vi "tpg361_visa_close.vi"(8 "error in (no error)":errorcluster, 11 "VISA session":refnum<visa-resource-name>) -> (0 "error out":errorcluster)   [LabVIEW 2019]
doc: "This VI closes the instrument.\n\nWARNINGS: \nYou MUSThave VISA Version 2.0 or higher installed to use this Instrument driver."
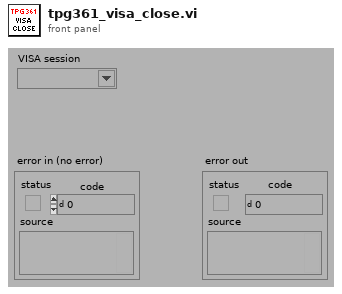
[diagram p1: front panel]
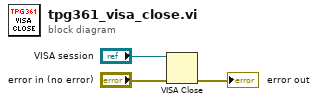
[diagram p0: block diagram]
diagram:
  n1 = VISA Close(VISA resource name="VISA session", error in (no error)="error in (no error)") -> (error out=→"error out":errorcluster)
